vi "FoodBox.vi"(7 "STOP":bool, 8 "Pellet in holder":bool=TRUE, 9 "Active":bool=TRUE, 10 "Max pellets":u32=2, 11 "ITI":u32=500) -> (2 "Number pellets":u32=500, 3 "Pellets taken":i32)   [LabVIEW 2021]
uses:
  <vilib>/DAQmx/write.llb/DAQmx Write (Digital Bool 1Line 1Point).vi
  <vilib>/DAQmx/create/channels.llb/DAQmx Create Channel (DO-Digital Output).vi
  GlobalSTATE.vi
  Global_BeamBreaks.vi
  <vilib>/DAQmx/miscellaneous.llb/DAQmx Fill In Error Info.vi
panel:
  out "TotalPelletsTaken":string
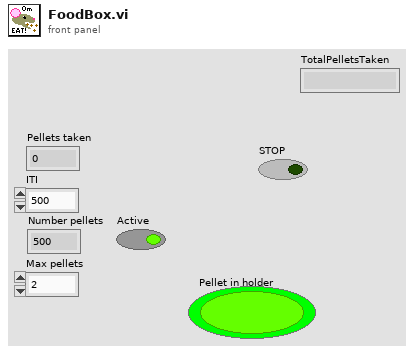
[diagram p1: front panel]
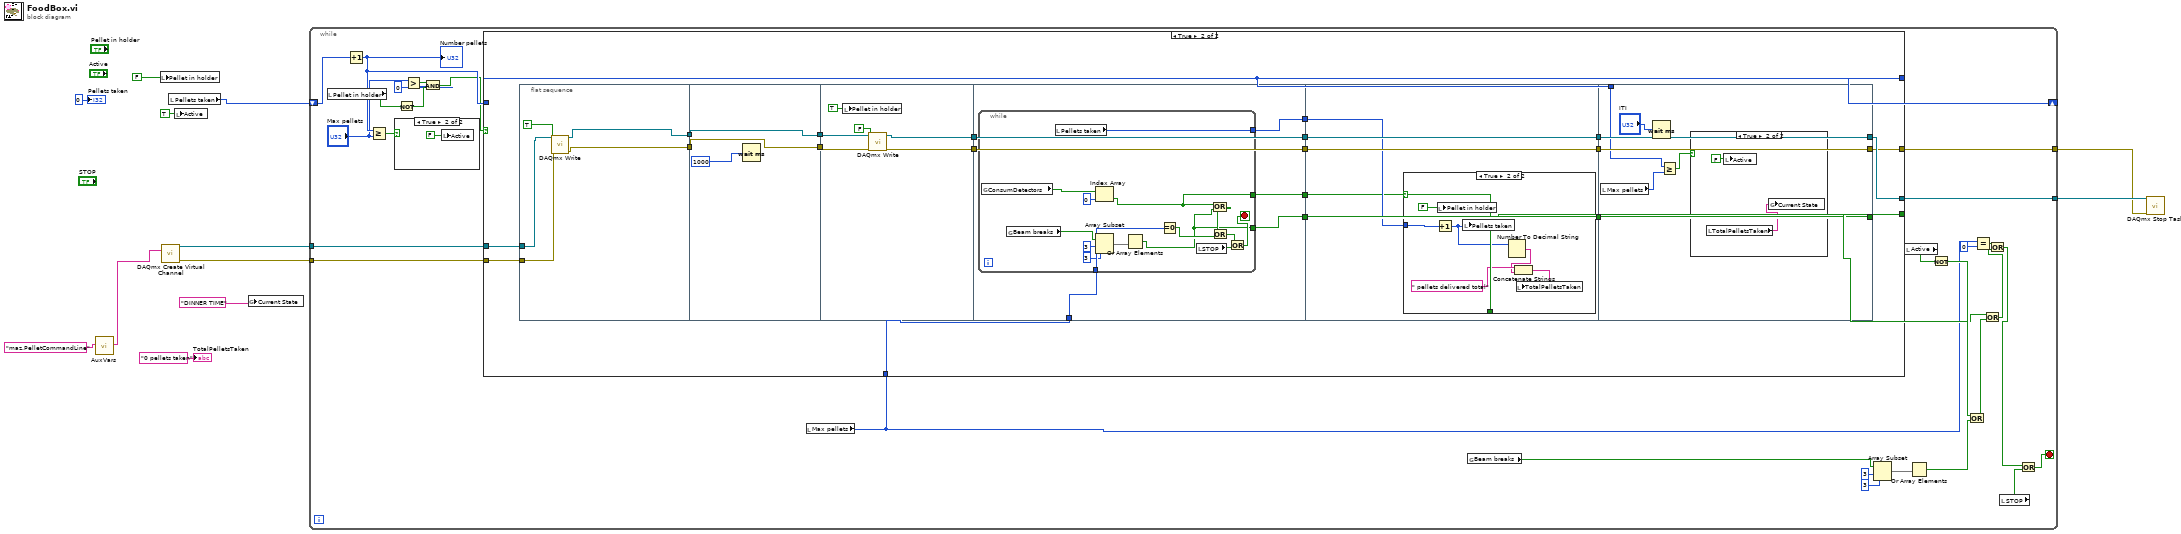
[diagram p0: block diagram]
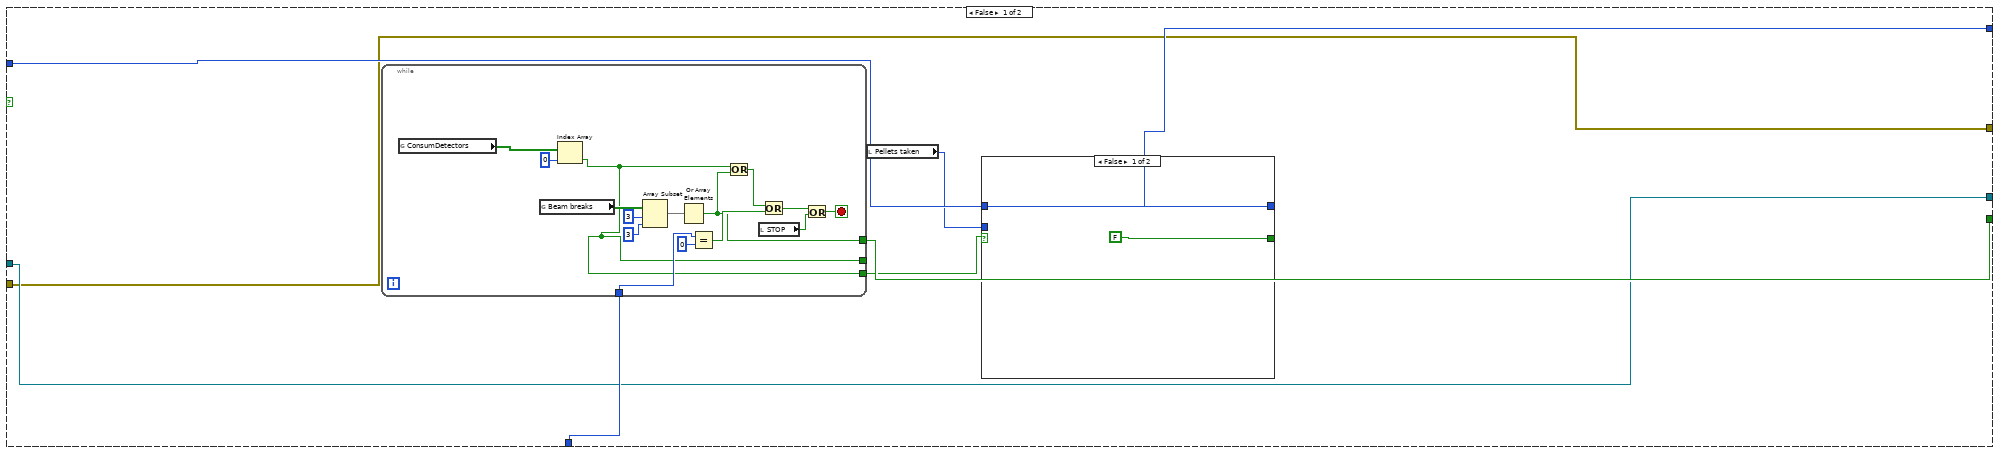
[diagram p3: hidden frame]
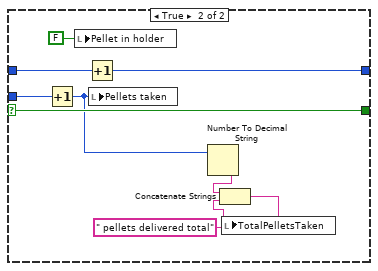
[diagram p4: hidden frame]
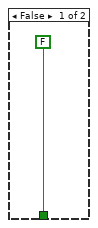
[diagram p5: hidden frame]
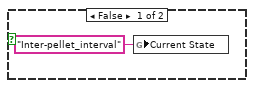
[diagram p6: hidden frame]
diagram:
  n1 = call "AuxVars.vi"("key"="maz.PelletCommandLine") -> ("value"=w9:string)  [unwired: 9 in, 1 out]
  n2 = local write "Pellet in holder"(FALSE ("Pellet in holder")) -> ()
  n3 = call-poly <vilib>:"DAQmx Create Virtual Channel.vi"("lines"=w9) -> ("task out"=w3:refnum<k21>, "error out"=w2:errorcluster)  [unwired: 13 in]
  n4 = local read "Pellets taken"() -> (w8:i32)
  n5 = local write "Active"(TRUE ("Active")) -> ()
  n6 = global write "GlobalSTATE.vi" "Current State"("DINNER TIME" ("Current State")) -> ()
  n7 = while {
    shift-right: [w41] -> _
    shift-left: w8 -> [w40]
    tunnel: [w16] -> w5
    tunnel: [w15] -> w4
    tunnel: w3 -> [w14]
    tunnel: w2 -> [w13]
    stop <- w22 stop-if-true
    n8 = local read "Pellet in holder"() -> (w42:bool)
    n9 = Increment(x=w40) -> (x+1=w37:i32)
    "Number pellets" <- w37
    n10 = Greater Or Equal?(x=w37, y="Max pellets") -> (x >= y?=w38:bool)
    n11 = case shown="True" w38 {
      frame False {
      }
      frame True {
        n12 = local write "Active"(FALSE ("Active")) -> ()
      }
    }
    n13 = Not(x=w42) -> (.not. x?=w30:bool)
    n14 = Greater?(x="Max pellets", y=u32 0) -> (0:w26:bool)
    n15 = And(x=w26, y=w30) -> (x .and. y?=w29:bool)
    n16 = local read "Max pellets"() -> (w25:u32)
    n17 = case shown="True" w29 {
      tunnel: w37 -> [w49 w92]
      tunnel: [w48 w92] -> w41
      tunnel: [w51 w91] -> w34
      tunnel: w25 -> [w50 w90]
      tunnel: [w45 w81] -> w16
      tunnel: [w44 w80] -> w15
      tunnel: w14 -> [w45 w79]
      tunnel: w13 -> [w44 w78]
      frame False {
        n18 = while {
          tunnel: [w66] -> w51
          tunnel: w50 -> [w76]
          tunnel: [w63] -> _
          tunnel: [w63] -> w46
          stop <- w71 stop-if-true
          n19 = global read "Global_BeamBreaks.vi" "ConsumDetectors"() -> (w65:bool[])
          n20 = global read "Global_BeamBreaks.vi" "Beam breaks"() -> (w68:bool[])
          n21 = Index Array(array=w65, index=0) -> (element=w63:bool)
          n22 = Array Subset(array=w68, index=3, length=3) -> (w67:bool[])
          n23 = Or Array Elements(Boolean array=w67) -> (logical OR=w66:bool)
          n24 = Equal?(x=w76, y=u32 0) -> (x = y?=w74:bool)
          n25 = Or(x=w63, y=w66) -> (x .or. y?=w77:bool)
          n26 = local read "STOP"() -> (w72:bool)
          n27 = Or(x=w77, y=w74) -> (x .or. y?=w73:bool)
          n28 = Or(x=w73, y=w72) -> (x .or. y?=w71:bool)
        }
        n29 = local read "Pellets taken"() -> (w47:i32)
        n30 = case shown="False" w46 {
          selector: w46 -> [_ w62]
          tunnel: [FALSE w62] -> _
          tunnel: w49 -> [w52 w60]
          tunnel: [w52 w59] -> w48
          tunnel: w47 -> [_ w58]
          frame False {
          }
          frame True {
            n31 = Increment(x=w58) -> (x+1=w54:i32)
            n32 = local write "Pellet in holder"(FALSE ("Pellet in holder")) -> ()
            n33 = Increment(x=w60) -> (x+1=w59:i32)
            n34 = local write "Pellets taken"(w54) -> ()
            n35 = Number To Decimal String(number=w54) -> (decimal integer string=w56:string)  [unwired: 1 in]
            n36 = Concatenate Strings(w56, " pellets delivered total" ("string")) -> (w57:string)
            n37 = local write "TotalPelletsTaken"(w57) -> ()
          }
        }
      }
      frame True {
        n38 = flat-sequence {
          tunnel: [w102] -> w98
          tunnel: [w101] -> w97
          tunnel: w79 -> [w100]
          tunnel: w78 -> [w99]
          tunnel: [w106] -> w96
          tunnel: w98 -> [w106]
          tunnel: [w105] -> w95
          tunnel: w97 -> [w105]
          tunnel: w96 -> [w111]
          tunnel: w95 -> [w110]
          tunnel: [w109] -> w94
          tunnel: [w108] -> w93
          tunnel: w94 -> [w118]
          tunnel: w93 -> [w117]
          tunnel: [w118] -> w89
          tunnel: [w117] -> w87
          tunnel: [w116] -> w85
          tunnel: w90 -> [w115]
          tunnel: [w114] -> w83
          tunnel: [w113] -> w82
          tunnel: w89 -> [w138]
          tunnel: [w138] -> w88
          tunnel: w87 -> [w137]
          tunnel: [w137] -> w86
          tunnel: w85 -> [w136]
          tunnel: [w136] -> w84
          tunnel: w83 -> [w135]
          tunnel: w82 -> [w134]
          tunnel: [w152] -> w80
          tunnel: [w153] -> w81
          tunnel: w88 -> [w153]
          tunnel: w86 -> [w152]
          tunnel: w92 -> [w147]
          tunnel: [w148] -> w91
          tunnel: w84 -> [w148]
          frame #0 {
            n39 = call-poly <vilib>:"DAQmx Write.vi"("task/channels in"=w100, "data"=TRUE, "error in"=w99) -> ("task out"=w102:refnum<k21>, "error out"=w101:errorcluster)  [unwired: 10 in, 1 out]
          }
          frame #1 {
            n40 = Wait (ms)(milliseconds to wait=u32 1000) -> ()  [unwired: 1 out]
          }
          frame #2 {
            n41 = local write "Pellet in holder"(TRUE ("Pellet in holder")) -> ()
            n42 = call-poly <vilib>:"DAQmx Write.vi"("task/channels in"=w111, "data"=FALSE, "error in"=w110) -> ("task out"=w109:refnum<k21>, "error out"=w108:errorcluster)  [unwired: 10 in, 1 out]
          }
          frame #3 {
            n43 = while {
              tunnel: [w123] -> w116
              tunnel: w115 -> [w133]
              tunnel: [w122] -> w114
              tunnel: [w119] -> w113
              stop <- w130 stop-if-true
              n44 = global read "Global_BeamBreaks.vi" "ConsumDetectors"() -> (w121:bool[])
              n45 = global read "Global_BeamBreaks.vi" "Beam breaks"() -> (w125:bool[])
              n46 = local read "Pellets taken"() -> (w122:i32)
              n47 = Index Array(array=w121, index=0) -> (element=w119:bool)
              n48 = Array Subset(array=w125, index=3, length=3) -> (w124:bool[])
              n49 = Or Array Elements(Boolean array=w124) -> (logical OR=w123:bool)
              n50 = Equal To 0?(x=w133) -> (x = 0?=w131:bool)
              n51 = local read "STOP"() -> (w128:bool)
              n52 = Or(x=w119, y=w123) -> (x .or. y?=w132:bool)
              n53 = Or(x=w132, y=w131) -> (x .or. y?=w129:bool)
              n54 = Or(x=w129, y=w128) -> (x .or. y?=w130:bool)
            }
          }
          frame #4 {
            n55 = case shown="True" w134 {
              selector: w134 -> [_ w146]
              tunnel: [FALSE w146] -> _
              tunnel: w135 -> [_ w144]
              frame False {
              }
              frame True {
                n56 = Increment(x=w144) -> (x+1=w143:i32)
                n57 = local write "Pellet in holder"(FALSE ("Pellet in holder")) -> ()
                n58 = local write "Pellets taken"(w143) -> ()
                n59 = Number To Decimal String(number=w143) -> (decimal integer string=w140:string)  [unwired: 1 in]
                n60 = Concatenate Strings(" pellets delivered total" ("string"), w140) -> (w142:string)
                n61 = local write "TotalPelletsTaken"(w142) -> ()
              }
            }
          }
          frame #5 {
            n62 = local read "Max pellets"() -> (w149:u32)
            n63 = Wait (ms)(milliseconds to wait="ITI") -> ()  [unwired: 1 out]
            n64 = Greater Or Equal?(x=w147, y=w149) -> (x >= y?=w150:bool)
            n65 = case shown="True" w150 {
              frame False {
                n66 = global write "GlobalSTATE.vi" "Current State"("Inter-pellet_interval" ("Current State")) -> ()
              }
              frame True {
                n67 = local read "TotalPelletsTaken"() -> (w155:string)
                n68 = local write "Active"(FALSE ("Active")) -> ()
                n69 = global write "GlobalSTATE.vi" "Current State"(w155) -> ()
              }
            }
          }
        }
      }
    }
    n70 = global read "Global_BeamBreaks.vi" "Beam breaks"() -> (w19:bool[])
    n71 = Array Subset(array=w19, index=3, length=3) -> (w18:bool[])
    n72 = local read "Active"() -> (w39:bool)
    n73 = Or Array Elements(Boolean array=w18) -> (logical OR=w17:bool)
    n74 = Not(x=w39) -> (.not. x?=w36:bool)
    n75 = Or(x=w36, y=w17) -> (x .or. y?=w35:bool)
    n76 = Equal?(x=w25, y=u32 0) -> (x = y?=w32:bool)
    n77 = Or(x=w34, y=w35) -> (x .or. y?=w33:bool)
    n78 = Or(x=w32, y=w33) -> (x .or. y?=w24:bool)
    n79 = local read "STOP"() -> (w23:bool)
    n80 = Or(x=w24, y=w23) -> (x .or. y?=w22:bool)
  }
  n81 = call <vilib>:"DAQmx Stop Task.vi"("task/channels in"=w5, "error in"=w4) -> ()  [unwired: 12 in, 2 out]
  "Pellets taken" <- 0 ("Pellets taken")
  "TotalPelletsTaken" <- "0 pellets taken" ("TotalPelletsTaken")
